vi "Constants.vi"() -> ()   [LabVIEW 2014, in "LVH-KinectOne.lvlib"]
uses:
  LVH-KinectOne.lvlib
panel:
  in  "InferredZPositionClamp":sgl=0.1
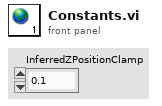
[diagram p1: front panel]
diagram:
